vi "GLOBALBridge.vi"() -> ()   [LabVIEW 2011]
panel:
  out "Bridge Output":dbl
  in  "Activitated":bool
  in  "Lower Limit":dbl=1.65
  in  "Upper Limit":dbl=3.8
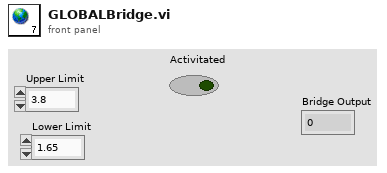
[diagram p1: front panel]
diagram:
